vi "Delay_MS_with_Error.vi"(8 "error in":errorcluster, 11 "delay before read (ms)":u32=500) -> (0 "error out":errorcluster)   [LabVIEW 2014]
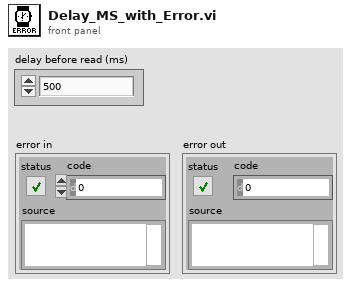
[diagram p1: front panel]
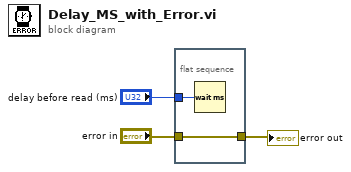
[diagram p0: block diagram]
diagram:
  n1 = flat-sequence {
    tunnel: "delay before read (ms)" -> [w5]
    tunnel: "error in" -> [w4]
    tunnel: [w4] -> w1
    frame #0 {
      n2 = Wait (ms)(milliseconds to wait=w5) -> ()  [unwired: 1 out]
    }
  }
  "error out" <- w1
